vi "SID_mem_to_voice.vi"(11 "mem":u8[](array[numeric]) format="%02x") -> (3 "VC":T1)   [LabVIEW 2018]
uses:
  SID_voice_reg.ctl
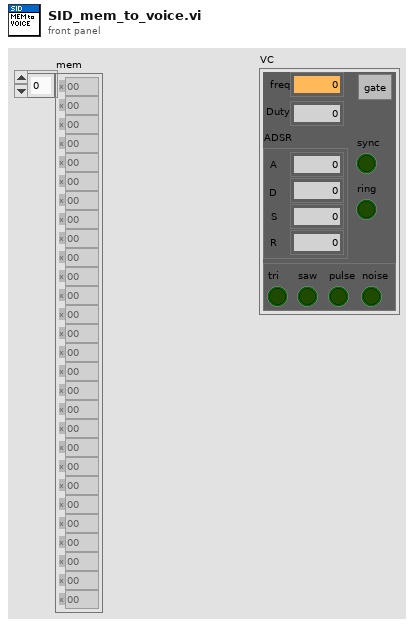
[diagram p1: front panel]
types:
  T1 = typedef "SID_voice_reg.ctl" = cluster{"freq":dbl, "gate":bool, "ADSR":cluster{"A":dbl, "D":dbl, "S":dbl, "R":dbl}, "Duty":dbl, "osc enab":cluster{"tri":bool, "saw":bool, "pulse":bool, "noise":bool}, "sync":bool, "ring":bool}
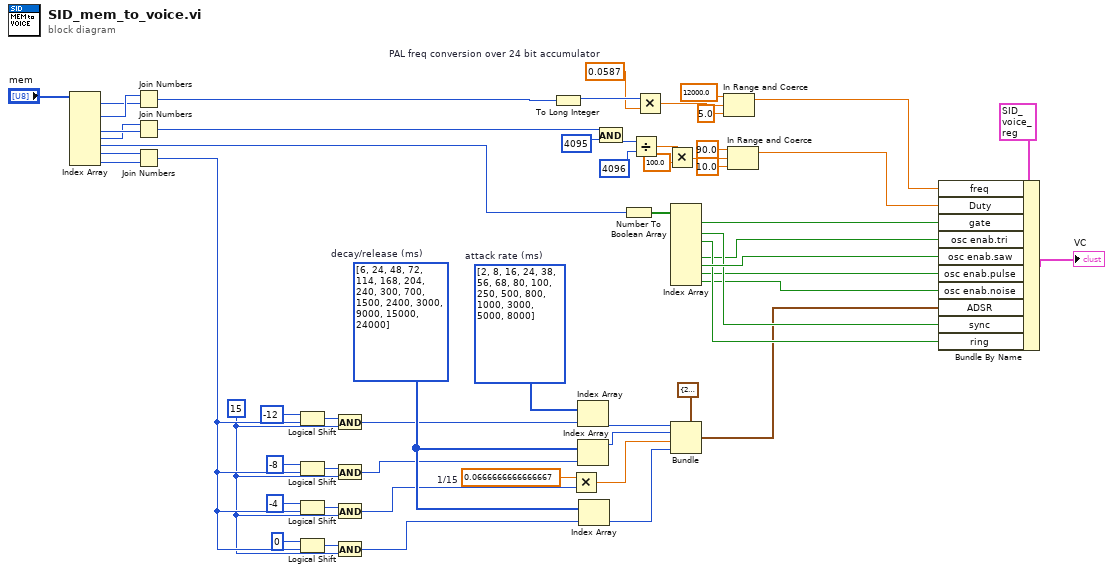
[diagram p0: block diagram]
diagram:
  w6 = u16 15 ("y")
  w19 = 0.0666666666666667  # 1/15
  w20 = 0.0587  # PAL freq conversion over 24 bit accumulator
  w46 = u16[] [6, 24, 48, 72, 114, 168, 204, 240, 300, 700, 1500, 2400, 3000, 9000, 15000, 24000]  # decay/release (ms)
  w47 = u16[] [2, 8, 16, 24, 38, 56, 68, 80, 100, 250, 500, 800, 1000, 3000, 5000, 8000]  # attack rate (ms)
  n1 = Index Array(array="mem") -> (element #1=w56:u8, element #2=w57:u8, element #3=w39:u8, element #4=w38:u8, element #5=w48:u8, element #6=w42:u8, element #7=w41:u8)  [unwired: 7 in]
  n2 = Join Numbers(hi=w57, lo=w56) -> ((hi.lo)=w55:u16)
  n3 = Join Numbers(hi=w38, lo=w39) -> ((hi.lo)=w34:u16)
  n4 = Join Numbers(hi=w42, lo=w41) -> ((hi.lo)=w7:u16)
  n5 = Logical Shift(y=i16 -12, x=w7) -> (x << y=w18:u16)
  n6 = Logical Shift(y=i16 -8, x=w7) -> (x << y=w14:u16)
  n7 = Logical Shift(y=i16 -4, x=w7) -> (x << y=w12:u16)
  n8 = Logical Shift(y=i16 0, x=w7) -> (x << y=w8:u16)
  n9 = And(x=w18, y=w6) -> (x .and. y?=w16:u16)
  n10 = And(x=w14, y=w6) -> (x .and. y?=w13:u16)
  n11 = And(x=w12, y=w6) -> (x .and. y?=w10:u16)
  n12 = And(x=w8, y=w6) -> (x .and. y?=w5:u16)
  n13 = To Long Integer(number=w55) -> (32bit integer=w21:i32)
  n14 = Multiply(x=w19, y=w10) -> (x*y=w22:dbl)
  n15 = Index Array(array=w47, index=w16) -> (element=w45:u16)
  n16 = Index Array(array=w46, index=w13) -> (element=w43:u16)
  n17 = Index Array(array=w46, index=w5) -> (element=w44:u16)
  n18 = And(x=w34, y=u16 4095) -> (x .and. y?=w32:u16)
  n19 = Number To Boolean Array(number=w48) -> (Boolean array=w54:bool[])
  n20 = Divide(x=w32, y=u16 4096) -> (x/y=w36:dbl)
  n21 = Multiply(x=w21, y=w20) -> (x*y=w2:dbl)
  n22 = Multiply(x=w36, y=100.0) -> (x*y=w24:dbl)
  n23 = Index Array(array=w54) -> (element #1=w27:bool, element #2=w52:bool, element #3=w51:bool, element #5=w40:bool, element #6=w53:bool, element #7=w29:bool, element #8=w28:bool)  [unwired: 8 in, 1 out]
  n24 = Bundle(cluster=cluster{"A":dbl, "D":dbl, "S":dbl, "R":dbl} {"A"=200.0, "D"=200.0, "S"=0.8, "R"=16.0} ("ADSR"), "A"=w45, "D"=w43, "S"=w22, "R"=w44) -> (w31:cluster{"A":dbl, "D":dbl, "S":dbl, "R":dbl})
  n25 = In Range and Coerce(upper limit=12000.0 ("y"), x=w2, lower limit=5.0) -> (coerced(x)=w1:dbl)  [unwired: 1 out]
  n26 = In Range and Coerce(upper limit=90.0, x=w24, lower limit=10.0) -> (coerced(x)=w23:dbl)  [unwired: 1 out]
  n27 = Bundle By Name(cluster=T1 {"freq"=0.0, "gate"=FALSE, "ADSR"={"A"=0.0, "D"=0.0, "S"=0.0, "R"=0.0}, "Duty"=0.0, "osc enab"={"tri"=FALSE, "saw"=FALSE, "pulse"=FALSE, "noise"=FALSE}, "sync"=FALSE, "ring"=FALSE} ("VC1"), "freq"=w1, "Duty"=w23, "gate"=w27, "osc enab.tri"=w40, "osc enab.saw"=w53, "osc enab.pulse"=w29, "osc enab.noise"=w28, "ADSR"=w31, "sync"=w52, "ring"=w51) -> (→"VC":T1)
